vi "Check_New_Devices.vi"(8 "error in (no error)":errorcluster) -> (0 "error out":errorcluster, 3 "Devices":refnum<visa-resource-name>[](array[refnum]))   [LabVIEW 2018]
uses:
  <resource>/objmgr/daqmx.rc
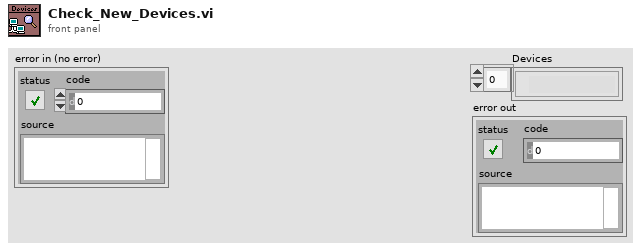
[diagram p1: front panel]
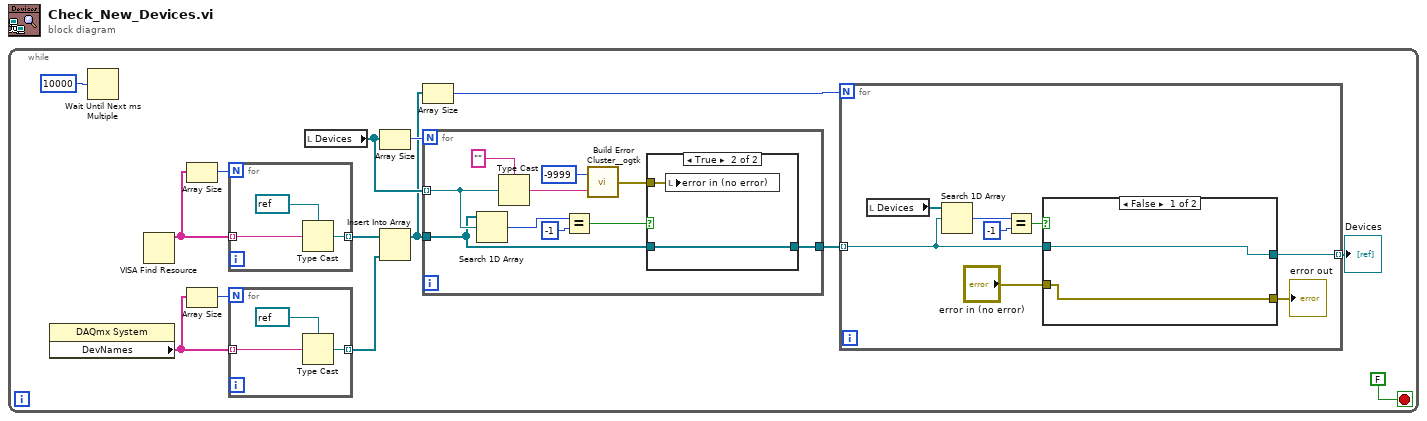
[diagram p0: block diagram]
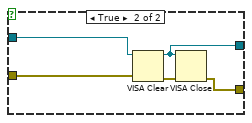
[diagram p3: hidden frame]
diagram:
  n1 = while {
    stop <- FALSE stop-if-true
    n2 = property class="DAQmx System"() -> ("DevNames"=w10:tag[])  [unwired: 2 in, 2 out]
    n3 = Wait Until Next ms Multiple(millisecond multiple=u32 10000) -> ()  [unwired: 1 out]
    n4 = VISA Find Resource() -> (3:w13:string[])  [unwired: 3 in, 2 out]
    n5 = Array Size(array=w13) -> (size(s)=w14:i32)
    n6 = Array Size(array=w10) -> (size(s)=w11:i32)
    n7 = for {
      N: w14 -> [_]
      tunnel: w13 -> [w48] mode=indexing
      tunnel: [w47] -> w12 mode=indexing
      n8 = Type Cast(type=refnum<visa-resource-name> refnum ("VISA resource name"), x=w48) -> (*(type *) &x=w47:refnum<visa-resource-name>)
    }
    n9 = for {
      N: w11 -> [_]
      tunnel: [w30] -> w9 mode=indexing
      tunnel: w10 -> [w28] mode=indexing
      n10 = Type Cast(type=refnum<visa-resource-name> refnum ("VISA resource name"), x=w28) -> (*(type *) &x=w30:refnum<visa-resource-name>)
    }
    n11 = local read "Devices"() -> (w3:refnum<visa-resource-name>[])
    n12 = Array Size(array=w3) -> (size(s)=w4:i32)
    n13 = Insert Into Array(array=w12, new element=w9) -> (w2:refnum<visa-resource-name>[])  [unwired: 1 in]
    n14 = Array Size(array=w2) -> (size(s)=w5:i32)
    n15 = for {
      N: w4 -> [_]
      tunnel: w3 -> [w21] mode=indexing
      tunnel: w2 -> [w16]
      tunnel: [w15] -> w1
      n16 = Search 1D Array(1D array=w16, element=w21) -> (index of element=w23:i32)  [unwired: 1 in]
      n17 = Type Cast(type="", x=w21) -> (*(type *) &x=w19:string)
      n18 = Equal?(x=w23, y=-1) -> (x = y?=w17:bool)
      n19 = call <userlib>:"Build Error Cluster__ogtk.vi"("String to Prepend to source (\"\")"=w19, "code"=-9999) -> ("error out"=w22:errorcluster)
      n20 = case shown="True" w17 {
        tunnel: w22 -> [_ w27]
        tunnel: w16 -> [w25 w26]
        tunnel: [w25 w26] -> w15
        frame False {
        }
        frame True {
          n21 = local write "error in (no error)"(w27) -> ()
        }
      }
    }
    n22 = for {
      N: w5 -> [_]
      tunnel: w1 -> [w34] mode=indexing
      tunnel: [w33] -> w8 mode=indexing
      n23 = local read "Devices"() -> (w35:refnum<visa-resource-name>[])
      n24 = Search 1D Array(1D array=w35, element=w34) -> (index of element=w38:i32)  [unwired: 1 in]
      n25 = Equal?(x=w38, y=-1) -> (x = y?=w36:bool)
      n26 = case shown="False" w36 {
        tunnel: w34 -> [w40 w45]
        tunnel: [w40 w44] -> w33
        tunnel: "error in (no error)" -> [w39 w42]
        tunnel: [w39 w41] -> w31
        frame False {
        }
        frame True {
          n27 = VISA Clear(VISA resource name=w45, error in (no error)=w42) -> (VISA resource name out=w44:refnum<visa-resource-name>, error out=w43:errorcluster)
          n28 = VISA Close(VISA resource name=w44, error in (no error)=w43) -> (error out=w41:errorcluster)
        }
      }
      "error out" <- w31
    }
    "Devices" <- w8
  }
